vi "参数簇转换字符串.vi"(10 "设置参数簇":T1) -> (2 "输入参数":string)   [LabVIEW 2015]
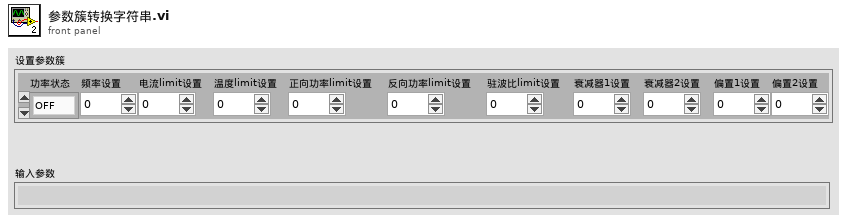
[diagram p1: front panel]
types:
  T1 = cluster{"功率状态":enum16{"OFF", "ON"}, "频率设置":dbl, "电流limit设置":u16, "温度limit设置":u16, "正向功率limit设置":u16, "反向功率limit设置":u16, "驻波比limit设置":u16, "衰减器1设置":u16, "衰减器2设置":u16, "偏置1设置":u16, "偏置2设置":u16}
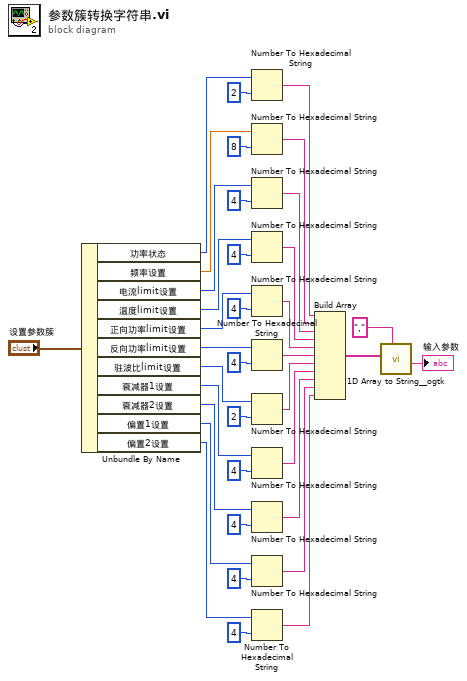
[diagram p0: block diagram]
diagram:
  n1 = Unbundle By Name("设置参数簇") -> ("功率状态"=w36:enum16{"OFF", "ON"}, "频率设置"=w34:dbl, "电流limit设置"=w31:u16, "温度limit设置"=w29:u16, "正向功率limit设置"=w27:u16, "反向功率limit设置"=w25:u16, "驻波比limit设置"=w23:u16, "衰减器1设置"=w18:u16, "衰减器2设置"=w17:u16, "偏置1设置"=w16:u16, "偏置2设置"=w15:u16)
  n2 = Number To Hexadecimal String(1:i16 2 ("宽度(-)"), 2:w36) -> (0:w14:string)
  n3 = Number To Hexadecimal String(1:i16 8 ("宽度(-)"), 2:w34) -> (0:w13:string)
  n4 = Number To Hexadecimal String(1:i16 4 ("宽度(-)"), 2:w31) -> (0:w12:string)
  n5 = Number To Hexadecimal String(1:i16 4 ("宽度(-)"), 2:w29) -> (0:w11:string)
  n6 = Number To Hexadecimal String(1:i16 4 ("宽度(-)"), 2:w27) -> (0:w10:string)
  n7 = Number To Hexadecimal String(1:i16 4 ("宽度(-)"), 2:w25) -> (0:w9:string)
  n8 = Number To Hexadecimal String(1:i16 2 ("宽度(-)"), 2:w23) -> (0:w8:string)
  n9 = Number To Hexadecimal String(1:i16 4 ("宽度(-)"), 2:w18) -> (0:w7:string)
  n10 = Number To Hexadecimal String(1:i16 4 ("宽度(-)"), 2:w17) -> (0:w6:string)
  n11 = Number To Hexadecimal String(1:i16 4 ("宽度(-)"), 2:w16) -> (0:w5:string)
  n12 = Number To Hexadecimal String(1:i16 4 ("宽度(-)"), 2:w15) -> (0:w4:string)
  n13 = Build Array(w14, w13, w12, w11, w10, w9, w8, w7, w6, w5, w4) -> (w3:string[])
  n14 = call <userlib>:"1D Array to String__ogtk.vi"("delimiter (Tab)"=",", "Array of Strings"=w3) -> ("delimited string"=→"输入参数":string)  [unwired: 9 in]
